vi "Process_And_Aim.vi"(0 "CameraDevRef":T3, 1 "Milsec Wait":u32=3000, 2 "Threshold Range":cluster{"Lower value":sgl, "Upper value":sgl}={"Lower value"=240.0, "Upper value"=255.0} {"Upper value" format="%.2f"; "Lower value" format="%.2f"}, 3 "Image Dsts Clust":T2) -> (20 "Offset Angle From Perpendicular":dbl, 21 "Shortest Dist To Rect Center":dbl, 22 "Image 1 Out":T1, 23 "Image 2 Out":T1, 24 "Binary 1 Out":T1, 25 "Binary 2 Out":T1, 26 "Processed Image Out":T1)   [LabVIEW 2011]
uses:
  <vilib>/Rock Robotics/WPI/Camera/WPI_CameraDevRef.ctl
  <vilib>/vision/Image Controls.llb/IMAQ Image.ctl
  <vilib>/Platform/TimedLoop/XDataNode/timing_clust.ctl
  <vilib>/Platform/TimedLoop/XDataNode/nitl_modes.ctl
  <vilib>/Platform/TimedLoop/XDataNode/wakeup.ctl
  <vilib>/Rock Robotics/WPI/Relay/WPI_RelayValue.ctl
  <vilib>/Platform/TimedLoop/XDataNode/XDataNode.xnode
  <vilib>/vision/NI_Vision_Development_Module.lvlib
  <vilib>/Platform/TimedLoop/XDataNode/XDNodeRunTimeDep.lvlib
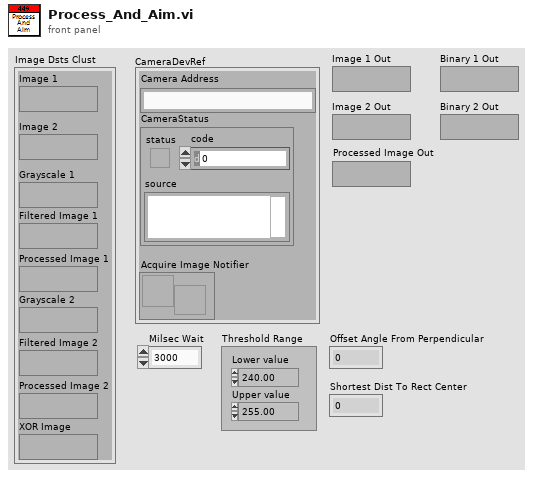
[diagram p1: front panel]
types:
  T1 = typedef "IMAQ Image.ctl" = refnum<image>
  T2 = cluster{"Image 1":T1, "Image 2":T1, "Grayscale 1":T1, "Filtered Image 1":T1, "Processed Image 1":T1, "Grayscale 2":T1, "Filtered Image 2":T1, "Processed Image 2":T1, "XOR Image":T1}
  T3 = typedef "WPI_CameraDevRef.ctl" = cluster{"Camera Address":string, "CameraStatus":errorcluster, "Acquire Image Notifier":refnum<notifier>}
  T4 = typedef "Image Type" = u32
  T5 = typedef "XDNodeRunTimeDep.lvlib/timing_clust.ctl" = cluster{"Expected End [f-1]":u64, "Actual End [f-1]":u64, "Finished Late? [f-1]":bool, "Expected End [i-1]":u64, "Actual End [i-1]":u64, "Finished Late? [i-1]":bool, "Expected Start [i]":u64, "Actual Start [i]":u64, "Expected Start [f]":u64, "Actual Start [f]":u64, "Source Name":string, "Structure Name":string, "Period":i64, "Deadline":i64, "Offset":i64, "Start":i64, "Priority":i32, "Timeout":i32, "Mode":T6, "Wakeup Reason":T7, "Error":errorcluster, "Source Type":string, "Secondary Source Type":string, "Global End Time":u64, "Global Start Time":u64, "Frame Duration":u64, "Iteration Duration":u64, "Assigned CPU":i32, "I/O Scan Engine Mode":u32}
  T6 = typedef "XDNodeRunTimeDep.lvlib/nitl_modes.ctl" = enum32{"No Change", "Process missed periods, maintain original phase", "Discard missed periods, maintain original phase", "Process missed periods, ignore original phase", "Discard missed periods, ignore original phase"}
  T7 = typedef "XDNodeRunTimeDep.lvlib/wakeup.ctl" = enum32{"Normal", "Aborted", "Asynchronous wakeup", "Timing source error", "Timed loop error", "Timeout"}
  T8 = typedef "WPI_RelayValue.ctl" = enum16{"Off", "On", "Forward", "Reverse"}
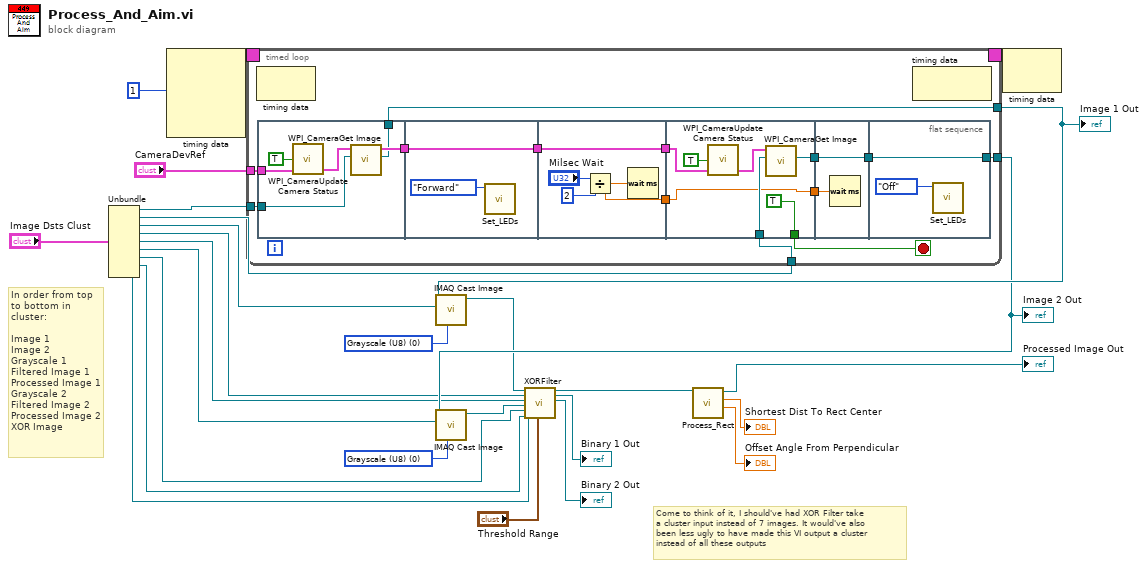
[diagram p0: block diagram]
diagram:
  w18 = T4 0 items=["Grayscale (U8)", "Grayscale (I16)", "Grayscale (SGL)", "Complex (CSG)", "RGB (U32)", "HSL (U32)", "RGB (U64)", "Grayscale (U16)"] ("Image Type")
  w19 = T4 0 items=["Grayscale (U8)", "Grayscale (I16)", "Grayscale (SGL)", "Complex (CSG)", "RGB (U32)", "HSL (U32)", "RGB (U64)", "Grayscale (U16)"] ("Image Type")
  # "Come to think of it, I should've had XOR Filter take\na cluster input instead of 7 images. It would've also\nbeen less ugly to have made this VI output a cluster\ninstead of all these outputs"
  # "In order from top\nto bottom in\ncluster:\n\nImage 1\nImage 2\nGrayscale 1\nFiltered Image 1\nProcessed Image 1\nGrayscale 2\nFiltered Image 2\nProcessed Image 2\nXOR Image"
  n1 = Unbundle("Image Dsts Clust") -> ("Image 1"=w17:T1, "Image 2"=w16:T1, "Grayscale 1"=w15:T1, "Filtered Image 1"=w9:T1, "Processed Image 1"=w8:T1, "Grayscale 2"=w13:T1, "Filtered Image 2"=w7:T1, "Processed Image 2"=w6:T1, "XOR Image"=w5:T1)
  n2 = node-c288(i64 1 ("Period")) -> (w27:T5)  [unwired: 3 in]
  n3 = timed-loop {
    tunnel: "CameraDevRef" -> [w39]
    tunnel: [w37] -> w12
    timing: w27 -> [_]
    timing-out: [_] -> w26
    tunnel: [w34] -> w14
    tunnel: w17 -> [w33]
    tunnel: w16 -> [w32]
    stop <- w38 stop-if-true
    n4 = node-c288() -> ()  [unwired: 1 in, 1 out]
    n5 = flat-sequence {
      tunnel: [w46] -> w36
      tunnel: w39 -> [w45]
      tunnel: [w44] -> w34
      tunnel: w33 -> [w43]
      tunnel: w36 -> [w50]
      tunnel: [w50] -> w35
      tunnel: [w54] -> w40
      tunnel: w35 -> [w54]
      tunnel: [w52] -> w28
      tunnel: w40 -> [w59]
      tunnel: [TRUE] -> w38
      tunnel: w32 -> [w56]
      tunnel: [w57] -> w31
      tunnel: [w55] -> w29
      tunnel: w28 -> [w55]
      tunnel: w31 -> [w63]
      tunnel: [w63] -> w30
      tunnel: w29 -> [w62]
      tunnel: [w65] -> w37
      tunnel: w30 -> [w65]
      frame #0 {
        n6 = call <vilib>:"WPI_CameraUpdate Camera Status.vi"("CameraDevRef In"=w45, "Enable Vision"=TRUE) -> ("CameraDevRef Out"=w48:T3)  [unwired: 3 in]
        n7 = call <vilib>:"WPI_CameraGet Image.vi"("Image"=w43, "CameraDevRef"=w48) -> ("Image Out"=w44:T1, "CameraDevRef Out"=w46:T3)  [unwired: 7 in, 1 out]
      }
      frame #1 {
        n8 = call "Set_LEDs.vi"("RelayValue"=WPI_RelayValue."Forward") -> ()  [unwired: 10 in, 1 out]
      }
      frame #2 {
        n9 = Divide(x="Milsec Wait", y=u32 2) -> (x/y=w52:dbl)
        n10 = Wait (ms)(milliseconds to wait=w52) -> ()  [unwired: 1 out]
      }
      frame #3 {
        n11 = call <vilib>:"WPI_CameraUpdate Camera Status.vi"("CameraDevRef In"=w59, "Enable Vision"=TRUE) -> ("CameraDevRef Out"=w60:T3)  [unwired: 3 in]
        n12 = call <vilib>:"WPI_CameraGet Image.vi"("Image"=w56, "CameraDevRef"=w60) -> ("Image Out"=w57:T1)  [unwired: 7 in, 2 out]
      }
      frame #4 {
        n13 = Wait (ms)(milliseconds to wait=w62) -> ()  [unwired: 1 out]
      }
      frame #5 {
        n14 = call "Set_LEDs.vi"("RelayValue"=WPI_RelayValue."Off") -> ()  [unwired: 10 in, 1 out]
      }
    }
    n15 = node-c288() -> ()  [unwired: 1 in, 1 out]
  }
  "Image 1 Out" <- w14
  "Image 2 Out" <- w12
  n16 = call "IMAQ Cast Image"("Image Type"=w19, "Image Dst"=w15, "Image Src"=w14) -> ("Image Dst Out"=w11:T1)  [unwired: 7 in, 1 out]
  n17 = call "IMAQ Cast Image"("Image Type"=w18, "Image Dst"=w13, "Image Src"=w12) -> ("Image Dst Out"=w10:T1)  [unwired: 7 in, 1 out]
  n18 = call "XORFilter.vi"("Image Src 1"=w11, "Filtered Image Dst 1"=w9, 2:"Processed Image Dst 2"=w8, "Image Src 2"=w10, "Filtered Image Dst 2"=w7, 5:"Processed Image Dst 2"=w6, "XOR Image Dst"=w5, "Threshold Range"="Threshold Range") -> ("XOR Image Dst Out"=w24:T1, "Image Dst 1 Out"=→"Binary 1 Out":T1, "Image Dst 2 Out"=→"Binary 2 Out":T1)  [unwired: 9 in]
  n19 = call "Process_Rect.vi"("XOR Image"=w24) -> ("Offset Angle From Perpendicular"=→"Offset Angle From Perpendicular":dbl, "Shortest Dist To Rect Center"=→"Shortest Dist To Rect Center":dbl, "Processed Image Out"=→"Processed Image Out":T1)  [unwired: 8 in]
  n20 = node-c288(w26) -> ()  [unwired: 1 out]
